vi "ECG Compression.vi"() -> ()   [LabVIEW 2023]
doc: "This example shows the application of the discrete wavelet transform (DWT) in signal compression.\n\nThe DWT transforms a signal into wavelet coefficients. The wavelet coefficients have most values close to zero. After quantizing the wavelet coefficients, you can set most of the coefficients to zero. So you can use entropy-based encoding techniques to reduce the bit rate of the wavelet coefficients and achieve signal compression.\n\nThis example uses the WA Discrete Wavelet Transform VI to transform an electrocardiogram (ECG) signal into wavelet coefficients and simulates the quantization for the wavelet coefficients. From the quantized wavelet coefficients, this example reconstructs the ECG signal using the WA Inverse Discrete Wavelet Transform VI and computes the signal to noise ratio (SNR) of the reconstructed signal. In real-world signal compression applications, you achieve compression by using entropy-based encoding techniques such as the Huffman coding to encode the quantized wavelet coefficients.\n\n<b>Instructions:</b>\n1) Run this VI.\n2) Change the number of <b>Bits</b> in the <b>Quantization</b> section to quantize the wavelet coefficients.\n3) Observe the <b>Compression Error</b> and <b>SNR (dB)</b>."
uses:
  <vilib>/addons/Wavelet Analysis/typedefs.llb/WA Data.ctl
  <vilib>/addons/Wavelet Analysis/discrete wavelet transform.llb/WA 1D Discrete Wavelet Transform (Array).vi
  <vilib>/addons/Wavelet Analysis/discrete wavelet transform.llb/WA Inverse 1D Discrete Wavelet Transform (Array).vi
  <vilib>/addons/_Advanced Signal Processing/NI_AdvSigProcWA.lvlib
panel:
  out "aspt-left-top":bool
  out "Compress Error":dbl[](graph)
  in  "stop":bool
  out "SNR (dB)":dbl
  in  "Bits":i32=8 min=1
  out "ECG":dbl[][](graph)
  in  "Levels":i32=11
  in  "Wavelet":u16(ring) items=["db02"=0, "db03"=1, "db04"=2, "db05"=3, "db06"=4, "db07"=5, "db08"=6, "db09"=7, "db10"=8, "db11"=9, "db12"=10, "db13"=11, "db14"=12, "Haar"=13, "bior1_3"=14, "bior1_5"=15, "bior2_2"=16, "bior2_4"=17, "bior2_6"=18, "bior2_8"=19, "bior3_1"=20, "bior3_3"=21, "bior3_5"=22, "bior3_7"=23, "bior3_9"=24, "bior4_4 (FBI)"=25, "bior5_5"=38, "bior6_8"=39, "coif1"=26, "coif2"=27, "coif3"=28, "coif4"=29, "coif5"=30, "sym2"=31, "sym3"=32, "sym4"=33, "sym5"=34, "sym6"=35, "sym7"=36, "sym8"=37]
  # "Overview: Shows the application of the discrete wavelet transform (DWT) in signal compression.\nRequirements: LabVIEW Full Development System, Advanced Signal Processing Toolkit\nInstructions: \n1. Run this VI.\n2. Change the number of Bits in the Quantization section to quantize the wavelet coefficients.\n3. Observe the Compression Error and SNR (dB).\n4. Click Stop to stop the VI."
  # "Wavelet Transform"
  # "Quantization"
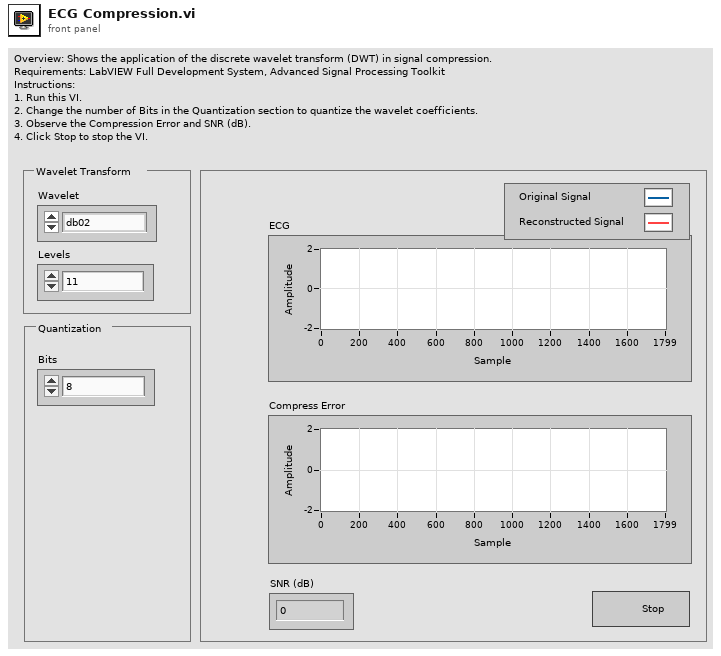
[diagram p1: front panel]
types:
  T1 = typedef "NI_AdvSigProcWA.lvlib/WA Data.ctl" = u16
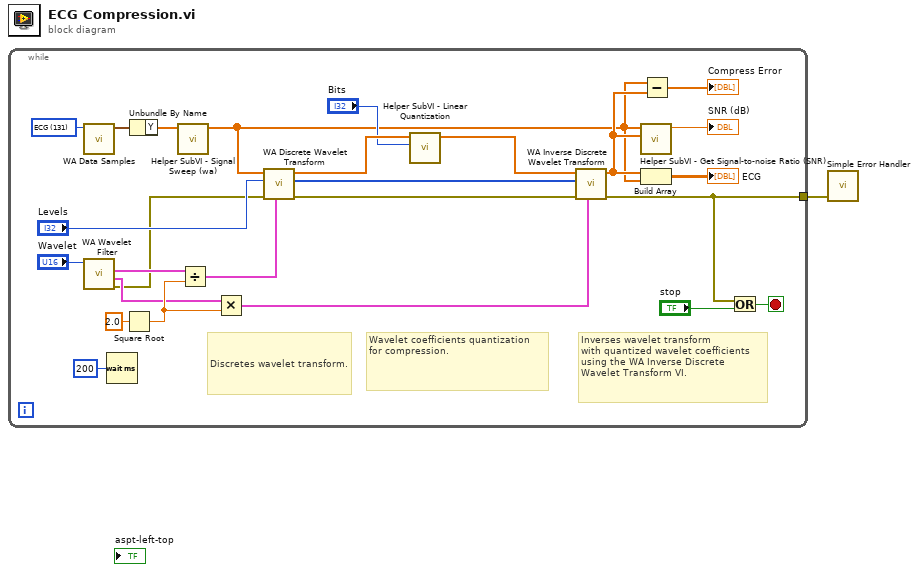
[diagram p0: block diagram]
diagram:
  n1 = while {
    tunnel: [w9] -> w1
    stop <- w17 stop-if-true
    w10 = T1 131 items=["1D Example Data"=100, "-"=101, "Doppler"=102, "HOP"=103, "TF Sine"=104, "Noisy Doppler"=105, "Sea Temperature"=106, "Sp500"=107, "Power Line"=108, "Engine Knocking"=109, "HeaviSine"=110, "Bumps"=111, "Blocks"=112, "Piece Regular"=113, "HypChirps"=114, "LinChirps"=115, "Chirps"=116, "Piece Polynomial"=117, "ECG"=131, "-"=118, "2D Example Data"=119, "-"=120, "Finger Print (Image)"=121, "Iris Flower (Image)"=122, "Mammogram (Image)"=123, "Lake (Image)"=127, "Two Can 1 (Image)"=132, "Two Can 2 (Image)"=133, "Camera Man (Image)"=134] ("data")
    # "Inverses wavelet transform \nwith quantized wavelet coefficients using the WA Inverse Discrete Wavelet Transform VI."
    # "Wavelet coefficients quantization \nfor compression."
    # "Discretes wavelet transform."
    n2 = call <vilib>:"WA Data Samples.vi"("data"=w10) -> ("signal"=w14:waveform(dbl))  [unwired: 10 out]
    n3 = call <vilib>:"WA Wavelet Filter.vi"("wavelet"="Wavelet") -> ("error out"=w8:errorcluster, "synthesis filters"=w12:cluster{"lowpass":dbl[], "highpass":dbl[]}, "analysis filters"=w24:cluster{"lowpass":dbl[], "highpass":dbl[]})  [unwired: 3 in, 5 out]
    n4 = Wait (ms)(milliseconds to wait=u32 200 ("millisecond multiple")) -> ()  [unwired: 1 out]
    n5 = Square Root(x=2.0) -> (sqrt(x)=w22:dbl)
    n6 = Unbundle By Name(w14) -> ("Y"=w13:dbl[])
    n7 = call "Helper SubVI - Signal Sweep (wa).vi"("Signal in"=w13) -> ("Signal out"=w2:dbl[])  [unwired: 10 in]
    n8 = Divide(x=w24, y=w22) -> (x/y=w20:cluster{"lowpass":dbl[], "highpass":dbl[]})
    n9 = Multiply(x=w12, y=w22) -> (x*y=w19:cluster{"lowpass":dbl[], "highpass":dbl[]})
    n10 = call-poly <vilib>:"WA Discrete Wavelet Transform.vi"("analysis filters"=w20, "error in (no error)"=w8, "levels"="Levels", "signal"=w2) -> ("error out"=w26:errorcluster, "length"=w27:i32[], "DWT coef"=w7:dbl[])  [unwired: 1 in, 4 out]
    n11 = call "Helper SubVI - Linear Quantization.vi"("bits"="Bits", "signal"=w7) -> ("quantized signal"=w5:dbl[])  [unwired: 9 in]
    n12 = call-poly <vilib>:"WA Inverse Discrete Wavelet Transform.vi"("synthesis filters"=w19, "error in (no error)"=w26, "length"=w27, "DWT coef"=w5) -> ("error out"=w9:errorcluster, "signal"=w3:dbl[])  [unwired: 1 in, 5 out]
    n13 = call "Helper SubVI - Get Signal-to-noise Ratio (SNR).vi"("noisy signal"=w3, "signal"=w2) -> ("SNR (dB)"=→"SNR (dB)":dbl)  [unwired: 9 in]
    n14 = Build Array(w3, w2) -> (→"ECG":dbl[][])
    n15 = Subtract(x=w2, y=w3) -> (x-y=→"Compress Error":dbl[])
    n16 = Or(x=w9, y="stop") -> (x .or. y?=w17:bool)
  }
  n17 = call <vilib>:"Simple Error Handler.vi"("error in (no error)"=w1) -> ()  [unwired: 1 in, 8 out]
